vi "4vs3 scale_ver11.vi"(0 "Input bitmap":i32[][](array[numeric])) -> (1 "Output bitmap":i32[][](array[numeric]), 2 "insert N":i32)   [LabVIEW 2016]
panel:
  out "Left, Top deleted(X, Y)":i32[](array[numeric])
  out "new picture 6":picture caption="fixed pic."
  out "Input bitmap 2":i32[][](array[numeric])
  out "Mid ¡/c ä":dbl
  out "Right, Bottom deleted(X, Y)":i32[](array[numeric])
  out "横/縦比":dbl format="%#_3g"
  out "pattern":u16
  out "new picture 4":picture caption="fixed pic."
  out "Output(X, Y)":i32[](array[numeric])
  out "Input (X, Y)":i32[](array[numeric])
  # "0 : equal\n1 :smaller(insert)\n2 : bigger(delete)"
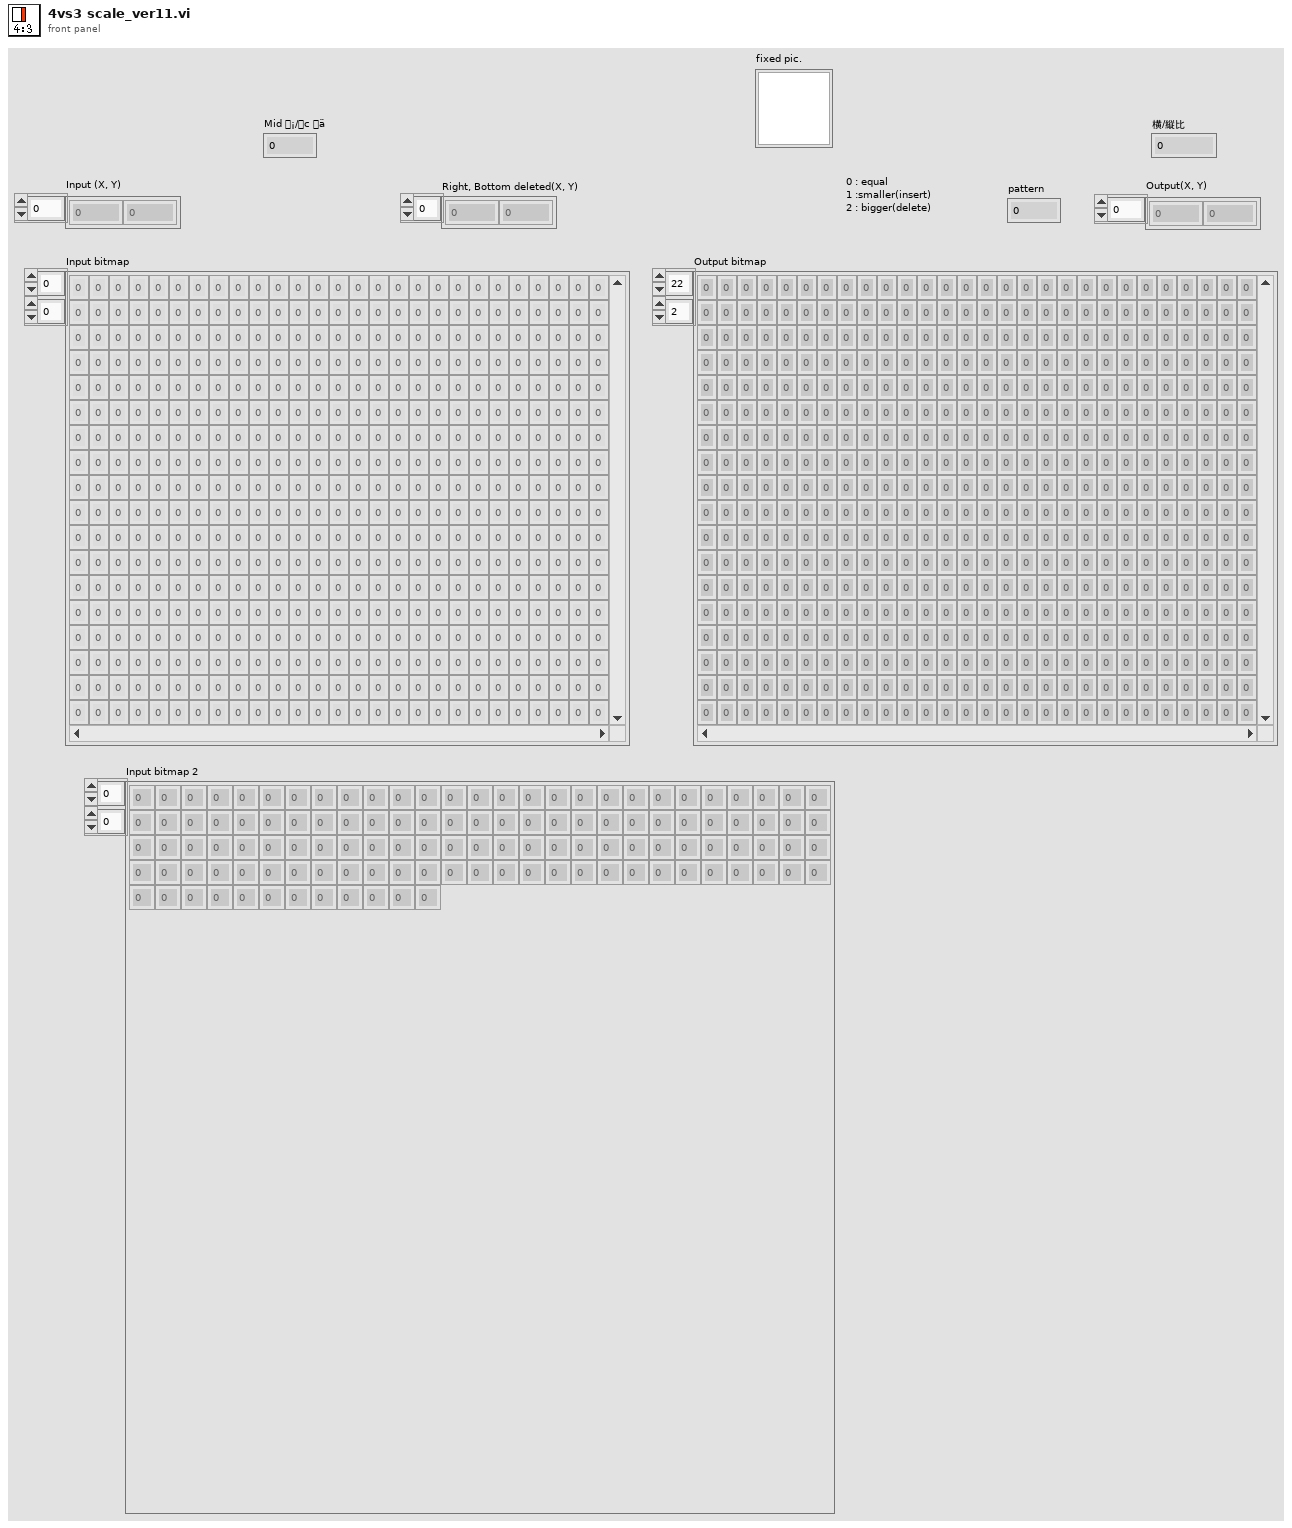
[diagram p1: front panel]
types:
  T1 = typedef "imagedata.ctl" = cluster{"image type":i32, "image depth":i32, "image":u8[], "mask":u8[], "colors":u32[], "Rectangle":cluster{"left":i16, "top":i16, "right":i16, "bottom":i16}}
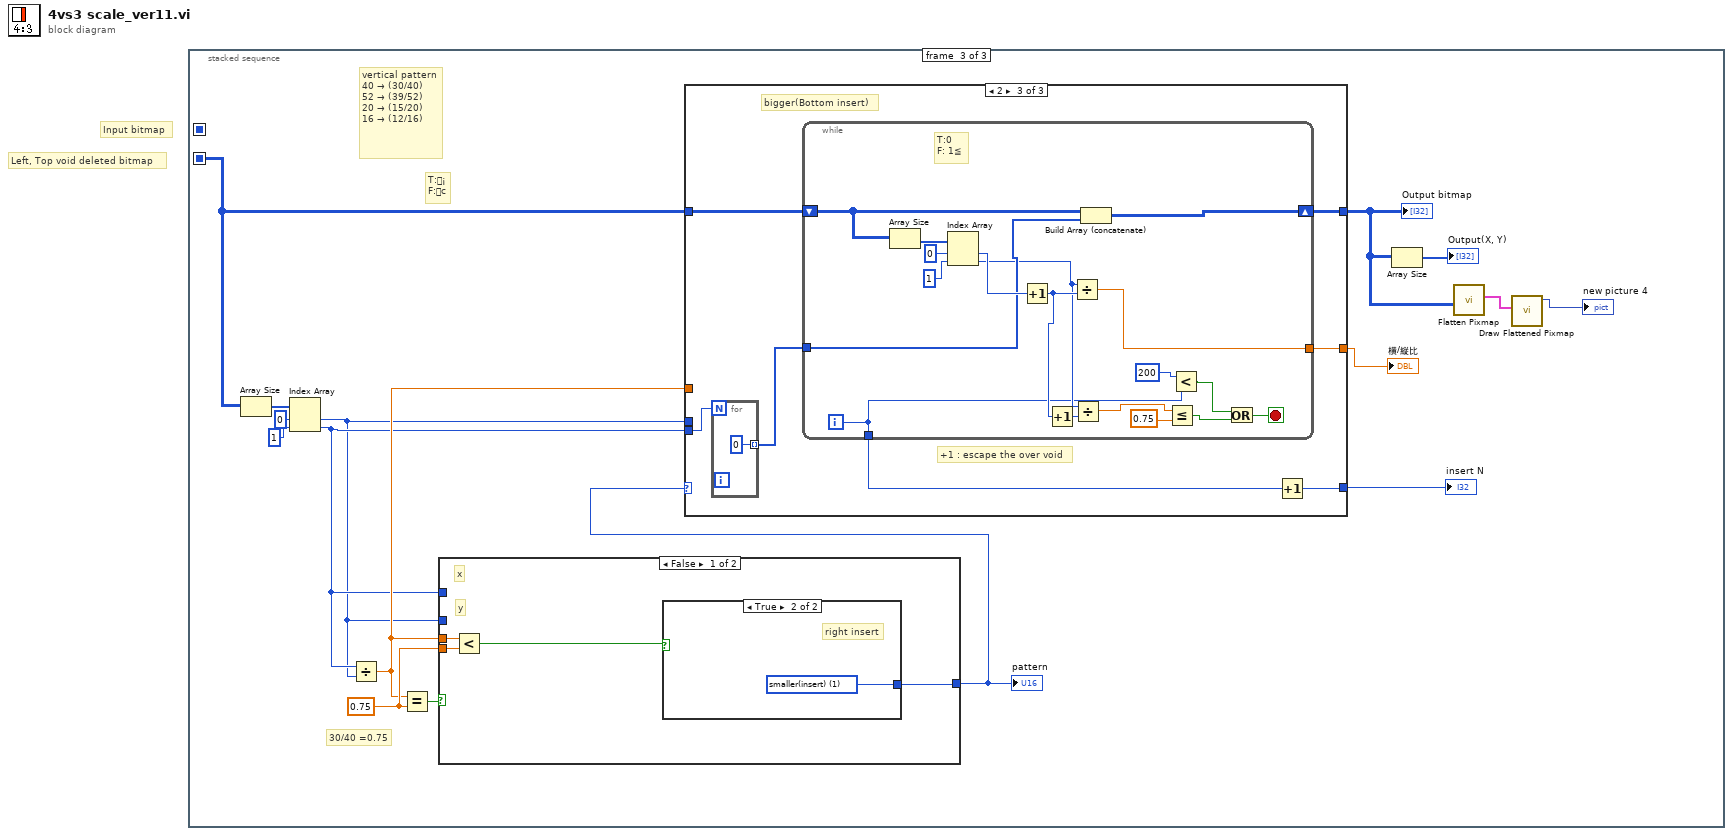
[diagram p0: block diagram]
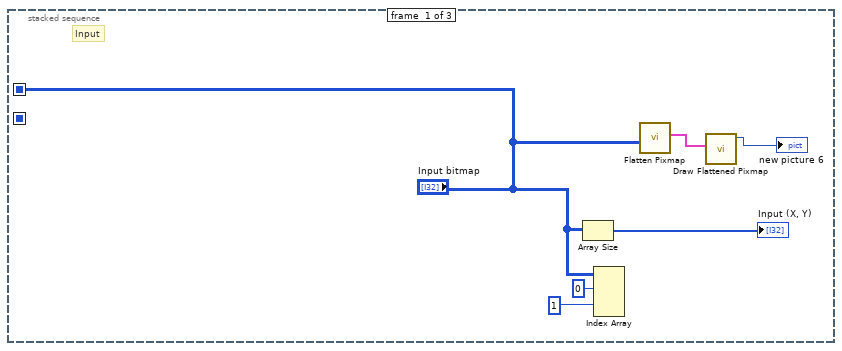
[diagram p2: hidden frame]
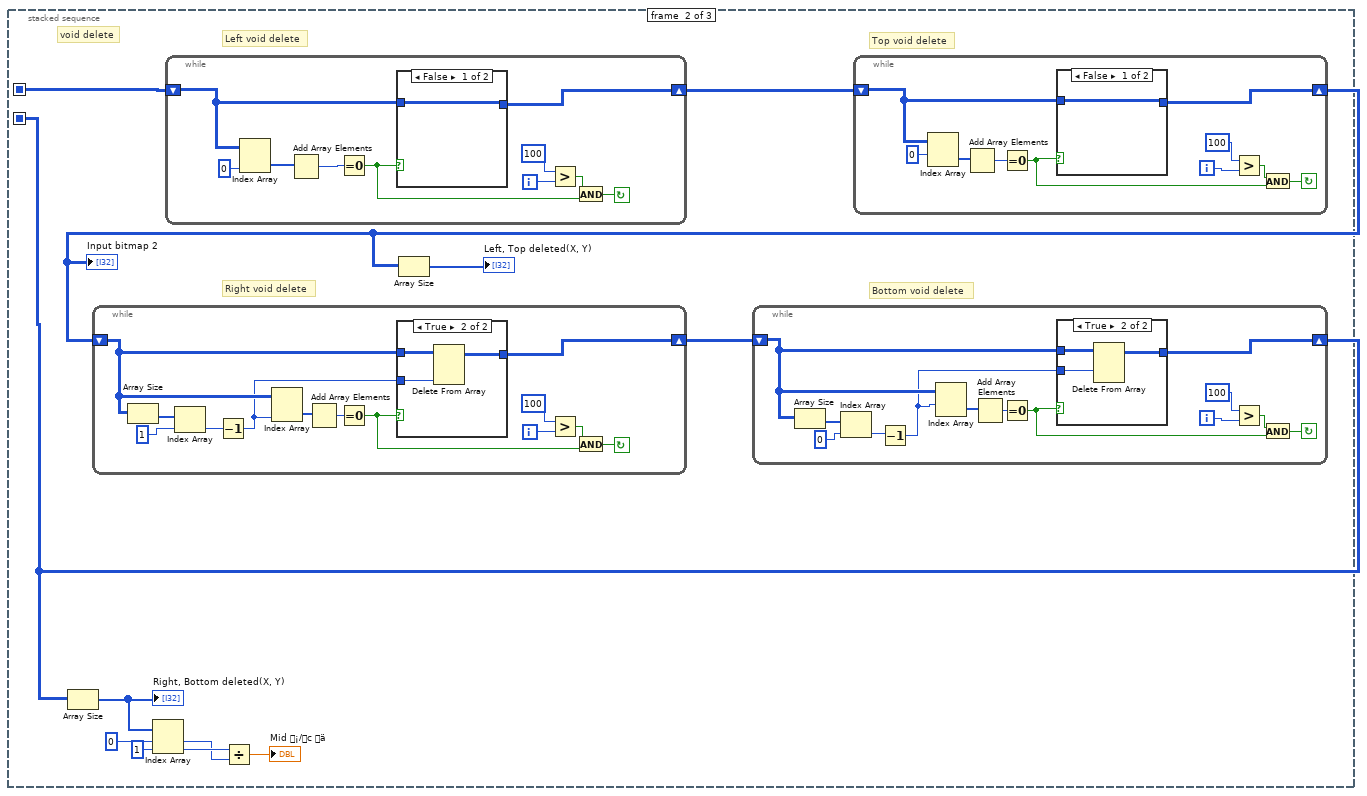
[diagram p3: hidden frame]
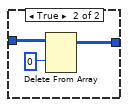
[diagram p6: hidden frame]
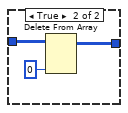
[diagram p7: hidden frame]
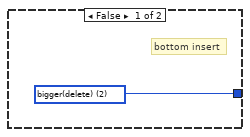
[diagram p8: hidden frame]
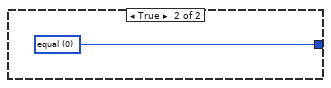
[diagram p9: hidden frame]
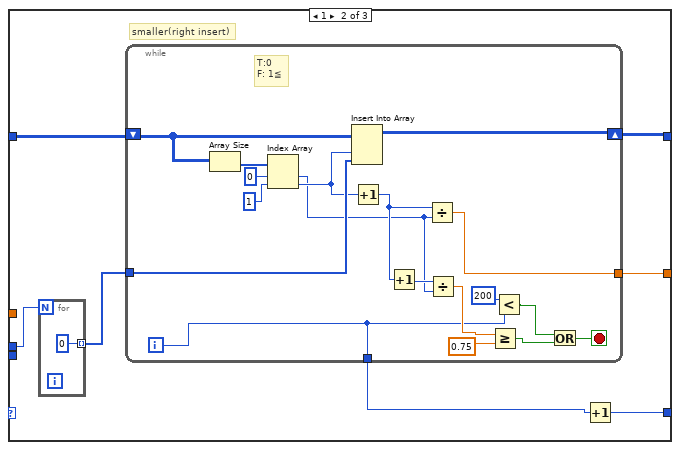
[diagram p11: hidden frame]
diagram:
  # "Left, Top void deleted bitmap"
  # "Input bitmap"
  n1 = stacked-sequence {
    seq-local: ["Input bitmap" _ _] -> [_ w18 _]
    seq-local: [_ w9 _] -> [_ _ w87]
    frame #0 {
      # "Input"
      n2 = Array Size(array="Input bitmap") -> (size(s)=→"Input (X, Y)":i32[])
      n3 = Index Array(array="Input bitmap", index (row) #1=0 ("指標"), index (row) #2=1) -> ()  [unwired: 2 in, 2 out]
      n4 = call <vilib>:"Flatten Pixmap.vi"("4-bit pixmap"="Input bitmap") -> ("image data"=w3:T1)  [unwired: 10 in]
      n5 = call <vilib>:"Draw Flattened Pixmap.vi"("image data"=w3) -> ("new picture"=→"new picture 6":picture)  [unwired: 8 in]
    }
    frame #1 {
      # "Bottom void delete"
      # "Right void delete"
      # "Top void delete"
      # "Left void delete"
      # "void delete"
      n6 = while {
        shift-right: [w72] -> w17
        shift-left: w18 -> [w73]
        i -> [w70]
        stop <- w69 continue-if-true
        n7 = Index Array(array=w73, index (col)=0 ("無効な指標 （列）")) -> (element=w76:i32[])  [unwired: 1 in]
        n8 = Add Array Elements(numeric array=w76) -> (sum=w75:i32)
        n9 = Equal To 0?(x=w75) -> (x = 0?=w67:bool)
        n10 = case shown="False" w67 {
          tunnel: w73 -> [w77 w80]
          tunnel: [w77 w78] -> w72
          frame False {
          }
          frame True {
            n11 = Delete From Array(array=w80, index (col)=0 ("無効な指標 （列）")) -> (array with subset deleted=w78:i32[][])  [unwired: 2 in, 1 out]
          }
        }
        n12 = Greater?(x=100, y=w70) -> (0:w68:bool)
        n13 = And(x=w68, y=w67) -> (x .and. y?=w69:bool)
      }
      n14 = while {
        shift-right: [w59] -> w7
        shift-left: w17 -> [w60]
        i -> [w56]
        stop <- w55 continue-if-true
        n15 = Index Array(array=w60, index (row)=0 ("無効な指標 （列）")) -> (element=w62:i32[])  [unwired: 1 in]
        n16 = Add Array Elements(numeric array=w62) -> (sum=w61:i32)
        n17 = Equal To 0?(x=w61) -> (x = 0?=w53:bool)
        n18 = case shown="False" w53 {
          tunnel: w60 -> [w63 w66]
          tunnel: [w63 w65] -> w59
          frame False {
          }
          frame True {
            n19 = Delete From Array(array=w66, index (row)=0 ("無効な指標 （列）")) -> (array with subset deleted=w65:i32[][])  [unwired: 2 in, 1 out]
          }
        }
        n20 = Greater?(x=100, y=w56) -> (0:w54:bool)
        n21 = And(x=w54, y=w53) -> (x .and. y?=w55:bool)
      }
      "Input bitmap 2" <- w7
      n22 = while {
        shift-right: [w46] -> w10
        shift-left: w7 -> [w40]
        i -> [w44]
        stop <- w43 continue-if-true
        n23 = Array Size(array=w40) -> (size(s)=w39:i32[])
        n24 = Index Array(array=w39, index=1 ("指標")) -> (element=w37:i32)
        n25 = Decrement(x=w37) -> (x-1=w36:i32)
        n26 = Index Array(array=w40, index (col)=w36) -> (element=w48:i32[])  [unwired: 1 in]
        n27 = Add Array Elements(numeric array=w48) -> (sum=w47:i32)
        n28 = Equal To 0?(x=w47) -> (x = 0?=w41:bool)
        n29 = case shown="True" w41 {
          tunnel: w40 -> [w49 w52]
          tunnel: [w49 w51] -> w46
          tunnel: w36 -> [_ w50]
          frame False {
          }
          frame True {
            n30 = Delete From Array(array=w52, index (col)=w50) -> (array with subset deleted=w51:i32[][])  [unwired: 2 in, 1 out]
          }
        }
        n31 = Greater?(x=100, y=w44) -> (0:w42:bool)
        n32 = And(x=w42, y=w41) -> (x .and. y?=w43:bool)
      }
      n33 = Array Size(array=w7) -> (size(s)=→"Left, Top deleted(X, Y)":i32[])
      n34 = while {
        shift-right: [w29] -> w9
        shift-left: w10 -> [w20]
        i -> [w27]
        stop <- w26 continue-if-true
        n35 = Array Size(array=w20) -> (size(s)=w23:i32[])
        n36 = Index Array(array=w23, index=0 ("指標")) -> (element=w21:i32)
        n37 = Decrement(x=w21) -> (x-1=w19:i32)
        n38 = Index Array(array=w20, index (row)=w19) -> (element=w31:i32[])  [unwired: 1 in]
        n39 = Add Array Elements(numeric array=w31) -> (sum=w30:i32)
        n40 = Equal To 0?(x=w30) -> (x = 0?=w24:bool)
        n41 = case shown="True" w24 {
          tunnel: w20 -> [w32 w35]
          tunnel: [w32 w34] -> w29
          tunnel: w19 -> [_ w33]
          frame False {
          }
          frame True {
            n42 = Delete From Array(array=w35, index (row)=w33) -> (array with subset deleted=w34:i32[][])  [unwired: 2 in, 1 out]
          }
        }
        n43 = Greater?(x=100, y=w27) -> (0:w25:bool)
        n44 = And(x=w25, y=w24) -> (x .and. y?=w26:bool)
      }
      n45 = Array Size(array=w9) -> (size(s)=w16:i32[])
      "Right, Bottom deleted(X, Y)" <- w16
      n46 = Index Array(array=w16, index #1=0 ("指標"), index #2=1 ("指標")) -> (element #1=w12:i32, element #2=w13:i32)
      n47 = Divide(x=w13, y=w12) -> (x/y=→"Mid ¡/c ä":dbl)
    }
    frame #2 {
      w96 = 0.75
      # "vertical pattern\n40 → (30/40)\n52 → (39/52)\n20 → (15/20)\n16 → (12/16)"
      # "30/40 =0.75"
      # "T:¡\nF:c"
      n48 = Array Size(array=w87) -> (size(s)=w90:i32[])
      n49 = Index Array(array=w90, index #1=0 ("指標"), index #2=1 ("指標")) -> (element #1=w82:i32, element #2=w83:i32)
      n50 = Divide(x=w83, y=w82) -> (x/y=w86:dbl)
      n51 = Equal?(x=w86, y=w96) -> (x = y?=w95:bool)
      n52 = case shown="False" w95 {
        tunnel: [w100 w103] -> w94
        tunnel: w96 -> [w98 _]
        tunnel: w86 -> [w97 _]
        tunnel: w83 -> [_ _]
        tunnel: w82 -> [_ _]
        frame False {
          # "y"
          # "x"
          n53 = Less?(x=w97, y=w98) -> (x < y?=w99:bool)
          n54 = case shown="True" w99 {
            tunnel: [w101 w102] -> w100
            frame False {
              w101 = u16 2 items=["equal", "smaller(insert)", "bigger(delete)", ""]
              # "bottom insert"
            }
            frame True {
              w102 = u16 1 items=["equal", "smaller(insert)", "bigger(delete)", ""]
              # "right insert"
            }
          }
        }
        frame True {
          w103 = u16 0 items=["equal", "smaller(insert)", "bigger(delete)", ""]
        }
      }
      "pattern" <- w94
      n55 = case shown="2" w94 {
        tunnel: w87 -> [w105 w112 w138]
        tunnel: [w105 w111 w137] -> w84
        tunnel: [w104 w110 w136] -> w85
        tunnel: w86 -> [w104 _ _]
        tunnel: w82 -> [_ w108 _]
        tunnel: w83 -> [_ _ w134]
        tunnel: [_ w106 w133] -> w81
        frame 0, Default {
        }
        frame 1 {
          # "smaller(right insert)"
          n56 = for {
            N: w108 -> [_]
            tunnel: [0] -> w109 mode=indexing
          }
          n57 = while {
            tunnel: w109 -> [w125]
            shift-right: [w120] -> w111
            shift-left: w112 -> [w124]
            tunnel: [w119] -> w110
            tunnel: [w114] -> w107
            i -> [w114]
            stop <- w128 stop-if-true
            # "T:0\nF: 1≦"
            n58 = Array Size(array=w124) -> (size(s)=w130:i32[])
            n59 = Index Array(array=w130, index #1=0, index #2=1) -> (element #1=w115:i32, element #2=w121:i32)
            n60 = Insert Into Array(array=w124, index (col)=w121, new element=w125) -> (w120:i32[][])  [unwired: 1 in]
            n61 = Increment(x=w121) -> (x+1=w117:i32)
            n62 = Increment(x=w117) -> (x+1=w116:i32)
            n63 = Divide(x=w117, y=w115) -> (x/y=w119:dbl)
            n64 = Divide(x=w116, y=w115) -> (x/y=w118:dbl)
            n65 = Greater Or Equal?(x=w118, y=0.75) -> (x >= y?=w129:bool)
            n66 = Less?(x=200, y=w114) -> (x < y?=w127:bool)
            n67 = Or(x=w127, y=w129) -> (x .or. y?=w128:bool)
          }
          n68 = Increment(x=w107) -> (x+1=w106:i32)
        }
        frame 2 {
          # "+1 : escape the over void"
          # "bigger(Bottom insert)"
          n69 = for {
            N: w134 -> [_]
            tunnel: [0] -> w135 mode=indexing
          }
          n70 = while {
            shift-right: [w148] -> w137
            shift-left: w138 -> [w151]
            tunnel: [w147] -> w136
            tunnel: w135 -> [w145]
            tunnel: [w140] -> w132
            i -> [w140]
            stop <- w154 stop-if-true
            # "T:0\nF: 1≦"
            n71 = Array Size(array=w151) -> (size(s)=w156:i32[])
            n72 = Index Array(array=w156, index #1=0, index #2=1) -> (element #1=w146:i32, element #2=w142:i32)
            n73 = Increment(x=w146) -> (x+1=w143:i32)
            n74 = Increment(x=w143) -> (x+1=w144:i32)
            n75 = Divide(x=w142, y=w143) -> (x/y=w147:dbl)
            n76 = Divide(x=w142, y=w144) -> (x/y=w141:dbl)
            n77 = Build Array (concatenate)(w151, w145) -> (w148:i32[][])
            n78 = Less Or Equal?(x=w141, y=0.75) -> (x <= y?=w155:bool)
            n79 = Less?(x=200, y=w140) -> (x < y?=w153:bool)
            n80 = Or(x=w153, y=w155) -> (x .or. y?=w154:bool)
          }
          n81 = Increment(x=w132) -> (x+1=w133:i32)
        }
      }
      "Output bitmap" <- w84
      "横/縦比" <- w85
      "insert N" <- w81
      n82 = Array Size(array=w84) -> (size(s)=→"Output(X, Y)":i32[])
      n83 = call <vilib>:"Flatten Pixmap.vi"("4-bit pixmap"=w84) -> ("image data"=w92:T1)  [unwired: 10 in]
      n84 = call <vilib>:"Draw Flattened Pixmap.vi"("image data"=w92) -> ("new picture"=→"new picture 4":picture)  [unwired: 8 in]
    }
  }
